vi "CheckWritePermission.vi"(6 "Method VI Name":string, 8 "error in (no error)":errorcluster, 11 "CS++Actor in":refnum<class "CS++Actor.lvclass">) -> (0 "error out":errorcluster, 3 "CS++Actor out":refnum<class "CS++Actor.lvclass">)   [LabVIEW 2016, in "CS++Actor.lvlib" / "CS++Actor.lvclass"]
uses:
  CS++Actor.lvclass
  CS++Actor.lvclass/CS++Actor.ctl
  <vilib>/ErrorRing/Error Ring.xnode
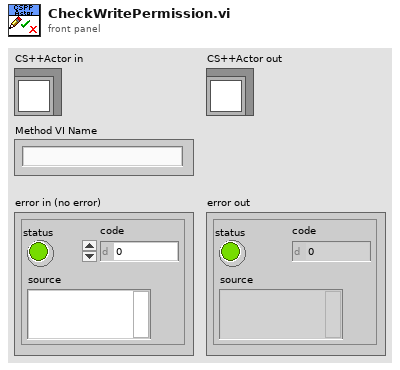
[diagram p1: front panel]
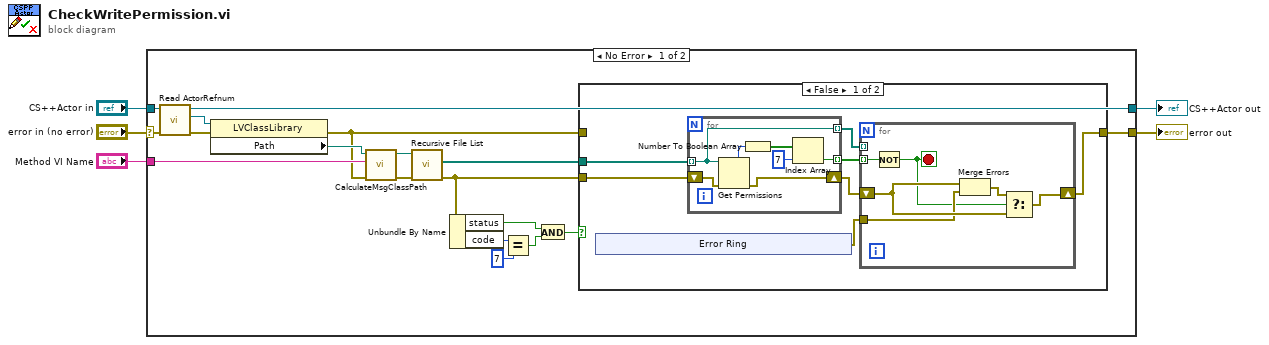
[diagram p0: block diagram]
diagram:
  n1 = case shown="No Error" "error in (no error)" {
    selector: "error in (no error)" -> [w20 w47]
    tunnel: [w22 w47] -> w4
    tunnel: [w19 w46] -> w2
    tunnel: "CS++Actor in" -> [w21 w46]
    tunnel: "Method VI Name" -> [w15 _]
    frame No Error {
      n2 = call "Read ActorRefnum.vi"("error in (no error)"=w20, "CS++Actor in"=w21) -> ("error out"=w18:errorcluster, "ActorRefnum"=w17:refnum<vi>, "CS++Actor out"=w19:refnum<class "CS++Actor.lvclass">)  [unwired: 7 in]
      n3 = property class="LVClassLibrary"(reference=w17, error in=w18) -> (error out=w6:errorcluster, "Path"=w16:path)  [unwired: 1 out]
      n4 = call "CalculateMsgClassPath.vi"("error in (no error)"=w6, "Method VI Name"=w15, "Actor Class Path"=w16) -> ("error out"=w14:errorcluster, "Message Class Path"=w13:path)  [unwired: 7 in]
      n5 = call <vilib>:"Recursive File List.vi"("error in (no error)"=w14, "Folder Path"=w13) -> ("error out"=w12:errorcluster, "All Files in Dir"=w23:path[])  [unwired: 5 in, 3 out]
      n6 = Unbundle By Name(w12) -> ("status"=w8:bool, "code"=w11:i32)
      n7 = Equal?(x=w11, y=7) -> (x = y?=w9:bool)
      n8 = And(x=w8, y=w9) -> (x .and. y?=w7:bool)
      n9 = case shown="False" w7 {
        tunnel: w23 -> [w30 _]
        tunnel: [w26 w45] -> w22
        tunnel: w12 -> [w24 _]
        tunnel: w6 -> [_ w45]
        frame False {
          n10 = xnode "Error Ring"() -> ("error out"=w25:errorcluster)
          n11 = for {
            tunnel: w30 -> [w37] mode=indexing
            shift-right: [w36] -> w27
            shift-left: w24 -> [w38]
            tunnel: [w32] -> w28 mode=indexing
            tunnel: [w37] -> w29 mode=indexing
            n12 = Get Permissions(8:w38, 11:w37) -> (0:w36:errorcluster, 5:w35:i16)  [unwired: 3 out]
            n13 = Number To Boolean Array(number=w35) -> (Boolean array=w34:bool[])
            n14 = Index Array(array=w34, index=7) -> (element=w32:bool)
          }
          n15 = for {
            tunnel: w29 -> [_] mode=indexing
            tunnel: w28 -> [w40] mode=indexing
            shift-right: [w41] -> w26
            shift-left: w27 -> [w43]
            tunnel: w25 -> [w42]
            stop <- w39 stop-if-true
            n16 = Not(x=w40) -> (.not. x?=w39:bool)
            n17 = Merge Errors(w43, w42) -> (w44:errorcluster)
            n18 = Select(t=w44, s=w39, f=w43) -> (s? t:f=w41:errorcluster)
          }
        }
        frame True {
        }
      }
    }
    frame Error {
    }
  }
  "error out" <- w4
  "CS++Actor out" <- w2
